vi "XML Root Token.vi"(10 "Tag":string, 11 "Namespace":string) -> (2 "Closing Item":string, 3 "Root Item":string)   [LabVIEW 2012]
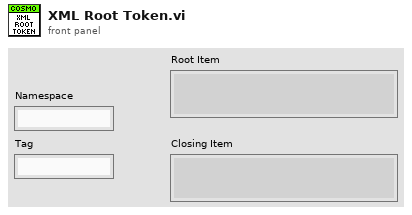
[diagram p1: front panel]
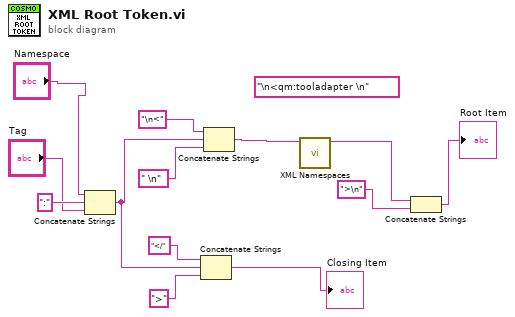
[diagram p0: block diagram]
diagram:
  (unwired) "\n<qm:tooladapter \n"
  n1 = Concatenate Strings("Namespace", ":" ("string"), "Tag") -> (w7:string)
  n2 = Concatenate Strings("</" ("string"), w7, ">" ("string")) -> (→"Closing Item":string)
  n3 = Concatenate Strings("\n<", w7, " \n") -> (w4:string)
  n4 = call "XML Namespaces.vi"("String in"=w4) -> ("String out"=w2:string)  [unwired: 10 in]
  n5 = Concatenate Strings(w2, ">\n") -> (→"Root Item":string)
